vi "Get Desired Size.vi"(8 "error in (no error)":errorcluster, 11 "Team Dashboard Panel in":refnum<class "Team Dashboard Panel.lvclass">) -> (0 "error out":errorcluster, 2 "Desired Size":T1, 3 "Team Dashboard Panel out":refnum<class "Team Dashboard Panel.lvclass">)   [LabVIEW 2020, in "SB App.lvlib" / "Team Dashboard Panel.lvclass"]
uses:
  Team Dashboard Panel.lvclass
  <vilib>/IlluminatedG/IG OOPanel/OOPanel/ArrayPanel/Desired Size.ctl
  <vilib>/IlluminatedG/IG OOPanel/OOPanel/OOPanel.lvlib
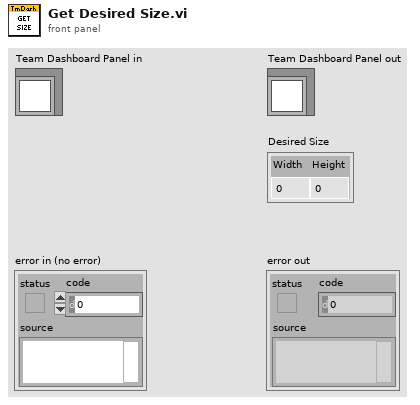
[diagram p1: front panel]
types:
  T1 = typedef "OOPanel.lvlib/Desired Size.ctl" = cluster{"Width":u32, "Height":u32}
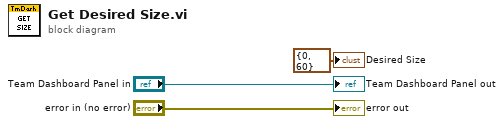
[diagram p0: block diagram]
diagram:
  "error out" <- "error in (no error)"
  "Team Dashboard Panel out" <- "Team Dashboard Panel in"
  "Desired Size" <- T1 {"Width"=0, "Height"=60} ("Desired Size")
